vi "IMAQ_Extract_Test.vi"() -> ()   [LabVIEW 2013]
uses:
  <vilib>/vision/Image Controls.llb/IMAQ Image.ctl
  <vilib>/vision/NI_Vision_Development_Module.lvlib
panel:
  out "Image Dst Out":T1
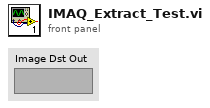
[diagram p1: front panel]
types:
  T1 = typedef "IMAQ Image.ctl" = refnum<image>
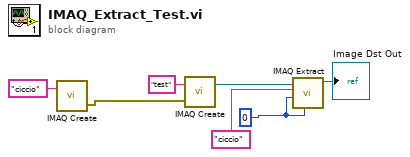
[diagram p0: block diagram]
diagram:
  w5 = 0
  n1 = call "IMAQ Create"("Image Name"="ciccio") -> ("error out"=w2:errorcluster)  [unwired: 4 in, 1 out]
  n2 = call "IMAQ Create"("Image Name"="test", "error in (no error)"=w2) -> ("New Image"=w6:T1)  [unwired: 3 in, 1 out]
  n3 = call "IMAQ Extract"("Y Step Size"=w5, "X Step Size"=w5, "Image Dst"="ciccio", "Image Src"=w6) -> ("Image Dst Out"=→"Image Dst Out":T1)  [unwired: 6 in, 1 out]
